vi "ProjectEditInterface.vi"(8 "error in (no error)":errorcluster, 11 "Project.lvclass In":refnum<class "Project.lvclass">) -> (0 "error out":errorcluster, 3 "Project.lvclass Out":refnum<class "Project.lvclass">)   [LabVIEW 2014, in "Project.lvclass"]
uses:
  Project.lvclass
panel:
  in  "ModifyStep":bool
  in  "RemoveStep":bool
  in  "AddStep":bool
  in  "StepList":i32(listbox)
  in  "ProjectList":i32(listbox)
  in  "RemoveProject":bool
  in  "AddProject":bool
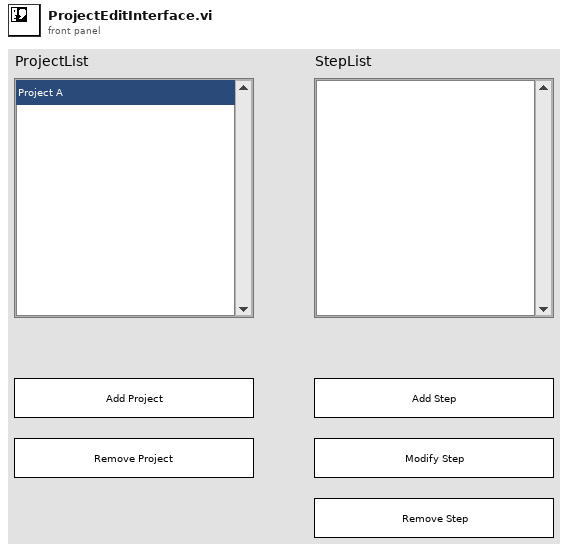
[diagram p1: front panel]
types:
  T1 = typedef "StepData.lvclass/StepTypeEnum.ctl" = enum16{"Move", "Measure"}
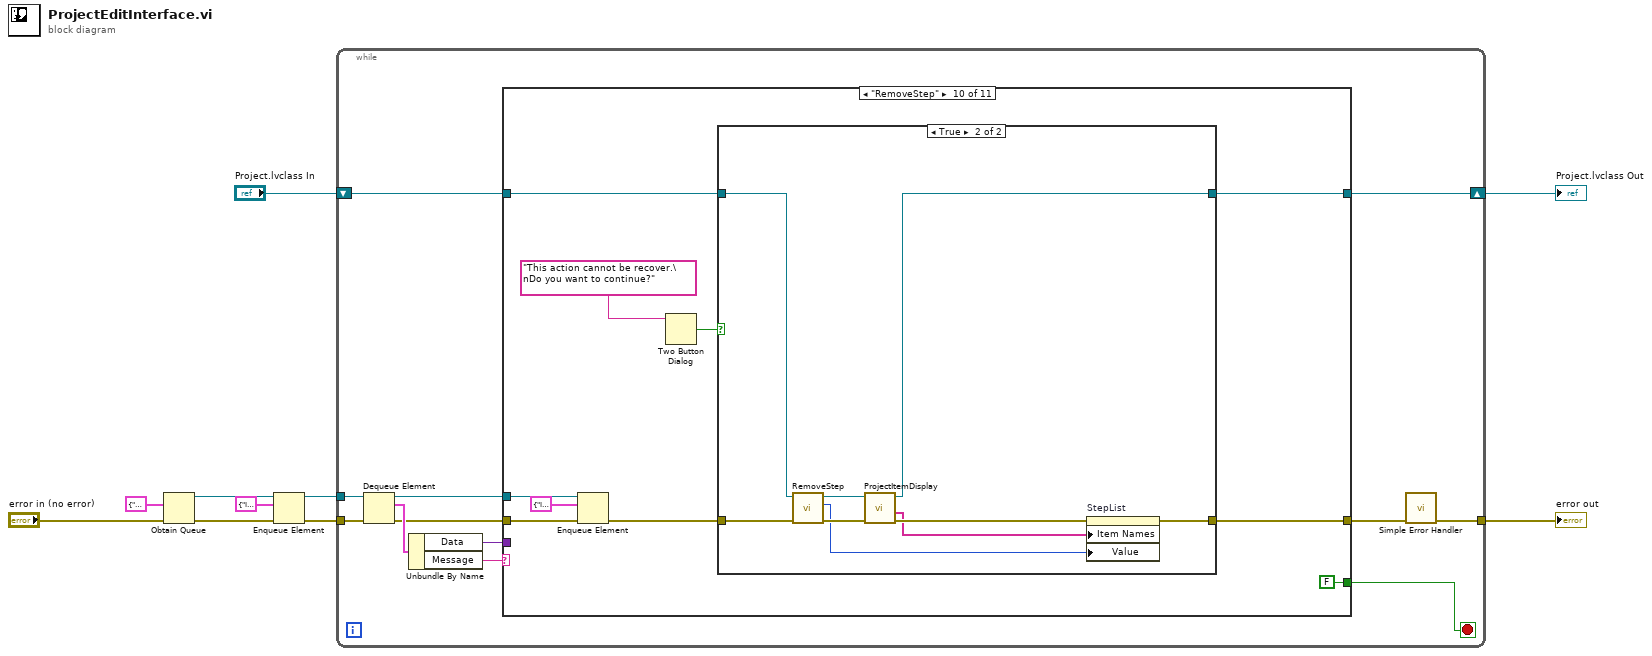
[diagram p0: block diagram]
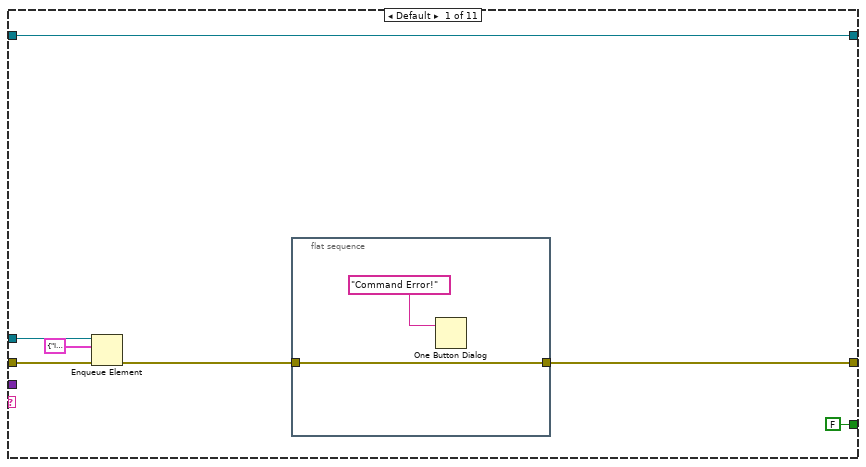
[diagram p2: hidden frame]
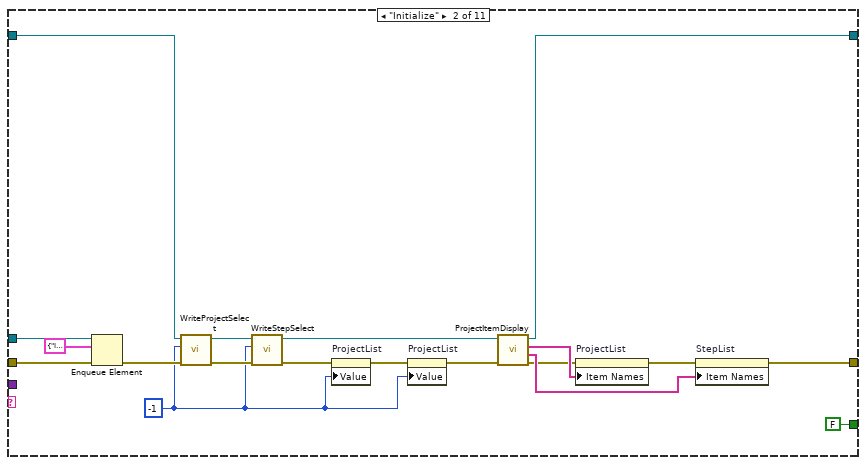
[diagram p3: hidden frame]
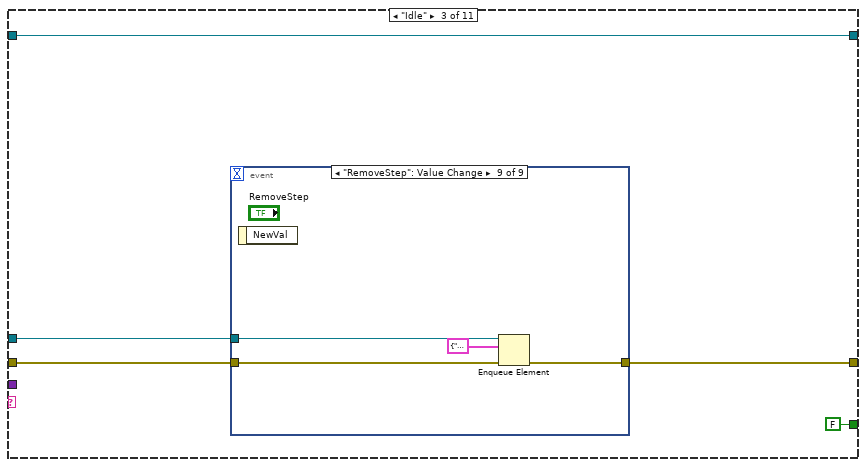
[diagram p4: hidden frame]
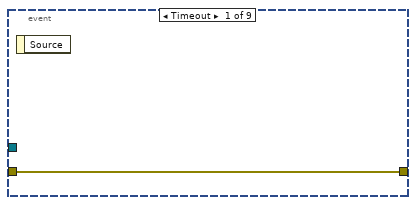
[diagram p5: hidden frame]
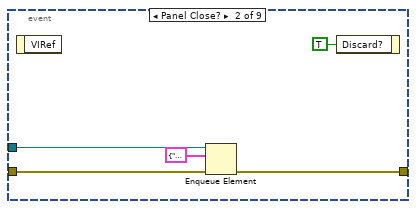
[diagram p6: hidden frame]
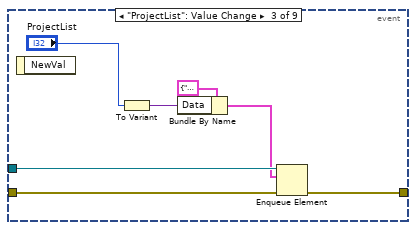
[diagram p7: hidden frame]
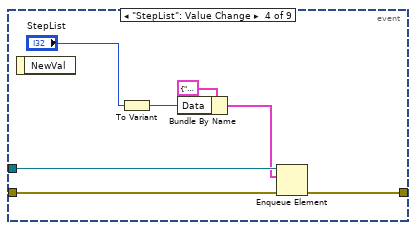
[diagram p8: hidden frame]
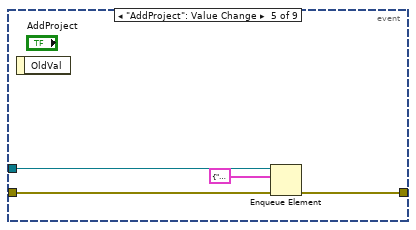
[diagram p9: hidden frame]
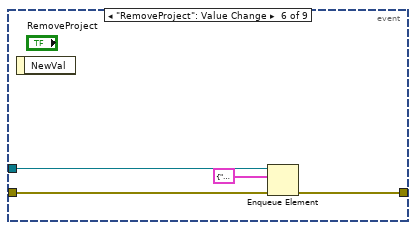
[diagram p10: hidden frame]
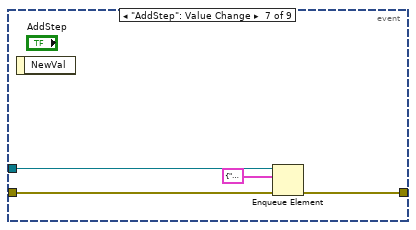
[diagram p11: hidden frame]
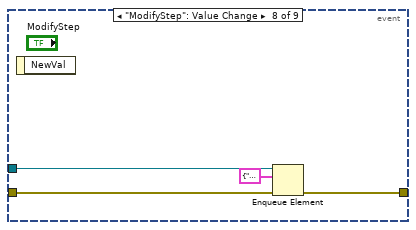
[diagram p12: hidden frame]
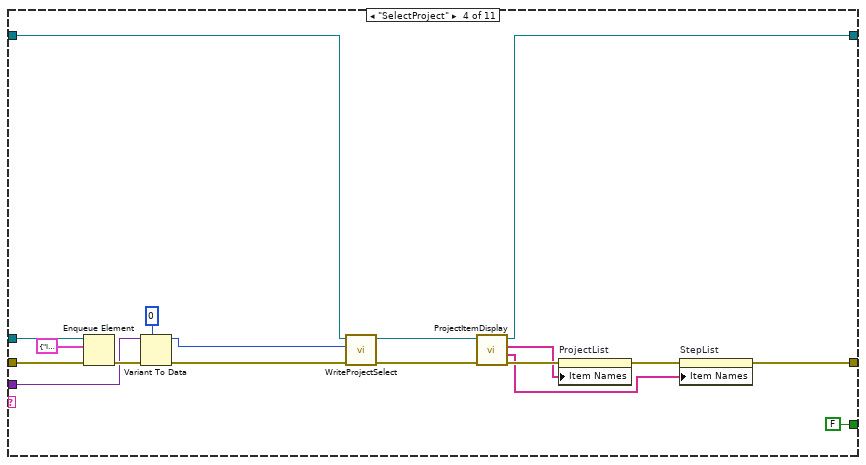
[diagram p13: hidden frame]
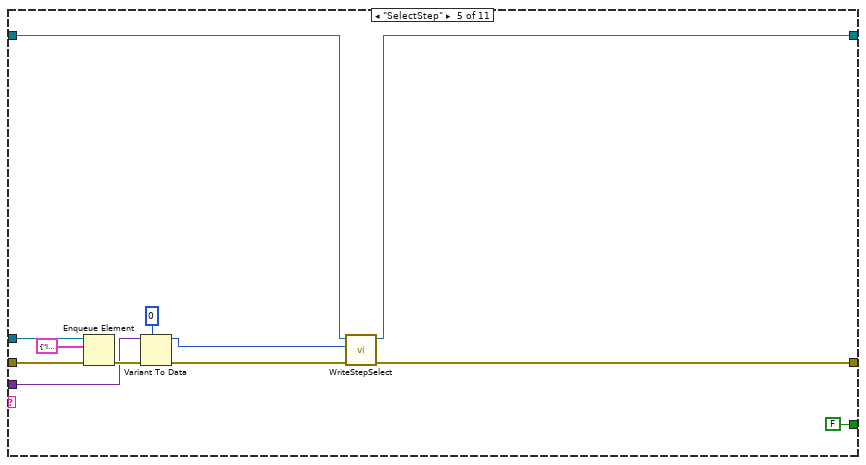
[diagram p14: hidden frame]
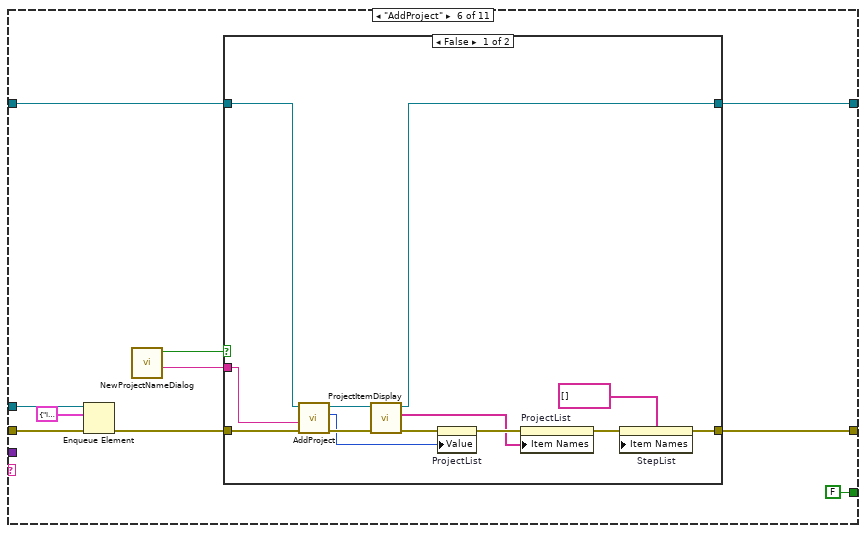
[diagram p15: hidden frame]
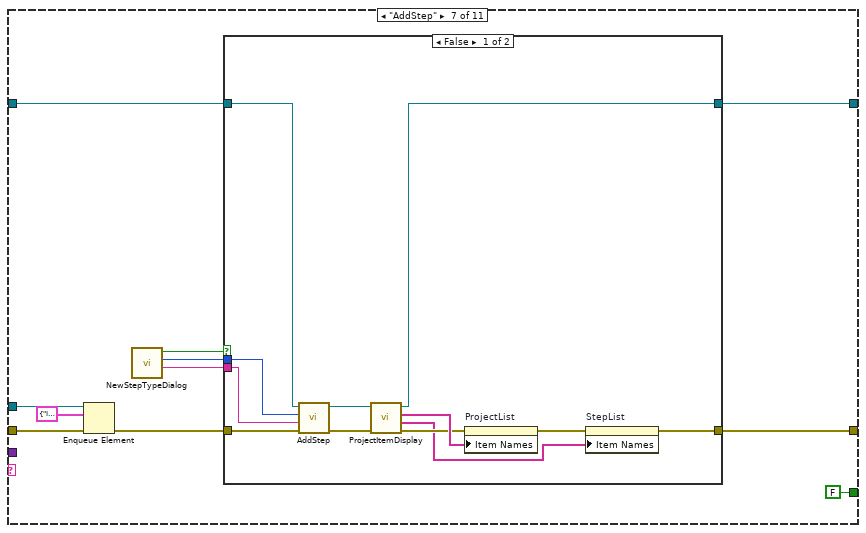
[diagram p17: hidden frame]
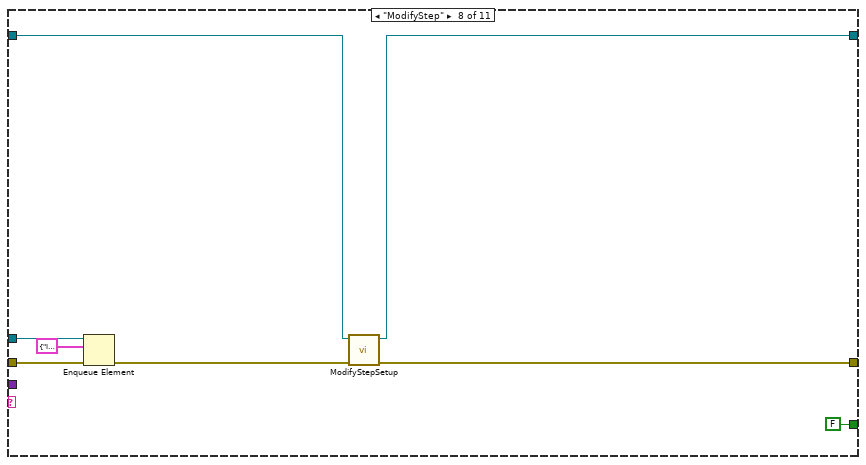
[diagram p19: hidden frame]
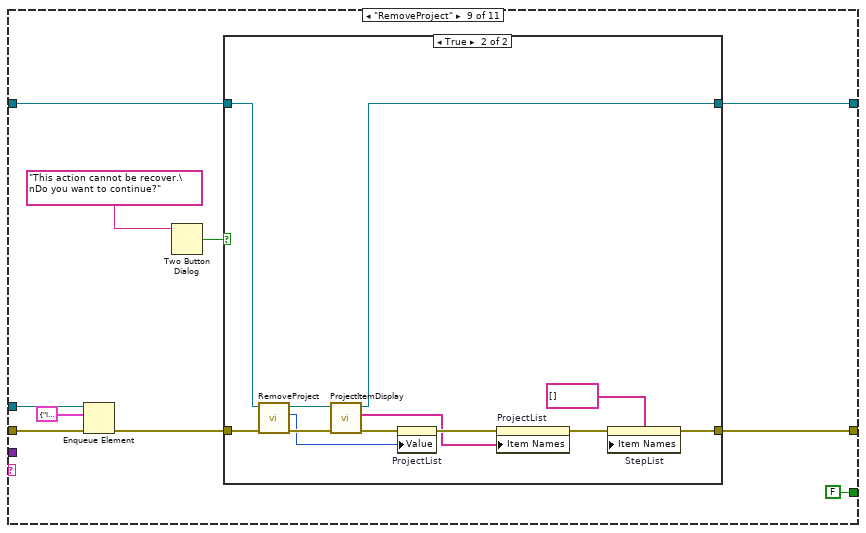
[diagram p20: hidden frame]
diagram:
  n1 = Obtain Queue(element data type=cluster{"Message":string, "Data":variant} {"Message"="", "Data"=variant}, error in (no error)="error in (no error)") -> (queue out=w9:refnum<queue>, error out=w10:errorcluster)  [unwired: 3 in, 1 out]
  n2 = Enqueue Element(queue=w9, element=cluster{"Message":string, "Data":variant} {"Message"="Initialize", "Data"=variant}, error in (no error)=w10) -> (queue out=w6:refnum<queue>, error out=w5:errorcluster)  [unwired: 1 in, 1 out]
  n3 = while {
    tunnel: w6 -> [w22]
    tunnel: w5 -> [w21]
    shift-right: [w14] -> w3
    shift-left: "Project.lvclass In" -> [w13]
    tunnel: [w11] -> w1
    stop <- w15 stop-if-true
    n4 = Dequeue Element(queue=w22, error in (no error)=w21) -> (queue out=w16:refnum<queue>, element=w20:cluster{"Message":string, "Data":variant}, error out=w18:errorcluster)  [unwired: 1 in, 1 out]
    n5 = Unbundle By Name(w20) -> ("Data"=w12:variant, "Message"=w19:string)
    n6 = case shown="\"RemoveStep\"" w19 {
      tunnel: w18 -> [w25 w50 w54 w113 w125 w135 w161 w183 w193 w217 w232]
      tunnel: [w29 w32 w53 w96 w114 w128 w156 w178 w188 w212 w230] -> w17
      tunnel: w16 -> [w23 w49 w55 w112 w124 w134 w160 w182 w192 w216 w231]
      tunnel: [FALSE FALSE FALSE FALSE FALSE FALSE FALSE FALSE FALSE FALSE TRUE] -> w15
      tunnel: [w27 w46 w51 w101 w115 w126 w154 w176 w184 w208 w229] -> w14
      tunnel: w13 -> [w27 w38 w51 w105 w117 w127 w155 w177 w185 w209 w229]
      tunnel: w12 -> [_ _ _ w108 w120 _ _ _ _ _ _]
      frame Default {
        n7 = Enqueue Element(queue=w23, element=cluster{"Message":string, "Data":variant} {"Message"="Idle", "Data"=variant}, error in (no error)=w25) -> (error out=w24:errorcluster)  [unwired: 1 in, 2 out]
        n8 = flat-sequence {
          tunnel: w24 -> [w31]
          tunnel: [w31] -> w29
          frame #0 {
            n9 = One Button Dialog(message="Command Error!") -> ()  [unwired: 1 in, 1 out]
          }
        }
      }
      frame "Initialize" {
        w36 = -1 ("ProjectList")
        n10 = Enqueue Element(queue=w49, element=cluster{"Message":string, "Data":variant} {"Message"="Idle", "Data"=variant}, error in (no error)=w50) -> (error out=w37:errorcluster)  [unwired: 1 in, 2 out]
        n11 = call "WriteProjectSelect.vi"("error in (no error)"=w37, "ProjectSelectIdx"=w36, "Project.lvclass In"=w38) -> ("error out"=w39:errorcluster, "Project.lvclass Out"=w40:refnum<class "Project.lvclass">)  [unwired: 7 in]
        n12 = call "WriteStepSelect.vi"("error in (no error)"=w39, "StepSelectIdx"=w36, "Project.lvclass In"=w40) -> ("error out"=w41:errorcluster, "Project.lvclass Out"=w42:refnum<class "Project.lvclass">)  [unwired: 7 in]
        n13 = property on="ProjectList" class="LstBox (strict)"(error in=w41, "Value"=w36) -> (error out=w44:errorcluster)  [unwired: 1 in, 1 out]
        n14 = property on="ProjectList" class="LstBox (strict)"(error in=w44, "Value"=w36) -> (error out=w43:errorcluster)  [unwired: 1 in, 1 out]
        n15 = call "ProjectItemDisplay.vi"("error in (no error)"=w43, "Project.lvclass In"=w42) -> ("error out"=w34:errorcluster, "StepNames"=w35:string[], "ProjectNames"=w45:string[], "Project.lvclass Out"=w46:refnum<class "Project.lvclass">)  [unwired: 5 in, 1 out]
        n16 = property on="ProjectList" class="LstBox (strict)"(error in=w34, "Item Names"=w45) -> (error out=w33:errorcluster)  [unwired: 1 in, 1 out]
        n17 = property on="StepList" class="LstBox (strict)"(error in=w33, "Item Names"=w35) -> (error out=w32:errorcluster)  [unwired: 1 in, 1 out]
      }
      frame "Idle" {
        n18 = event shown="[8] \"RemoveStep\": Value Change" {
          selector: _ -> [_ _ _ _ _ _ _ _ _]
          dyn-events: _ -> [_ _ _ _ _ _ _ _ _]
          timeout: _ -> [_ _ _ _ _ _ _ _ _]
          tunnel: w55 -> [_ w58 w66 w73 w78 w82 w85 w89 w93]
          tunnel: w54 -> [w56 w60 w68 w75 w79 w83 w87 w91 w95]
          tunnel: [w56 w59 w67 w74 w77 w81 w86 w90 w94] -> w53
          event Timeout {
            n19 = event-data() -> ()  [unwired: 1 in, 1 out]
          }
          event Panel Close? {
            n20 = event-data() -> ()  [unwired: 1 in, 1 out]
            n21 = Enqueue Element(queue=w58, element=cluster{"Message":string, "Data":variant} {"Message"="Exit", "Data"=variant}, error in (no error)=w60) -> (error out=w59:errorcluster)  [unwired: 1 in, 2 out]
            n22 = event-data("Discard?"=TRUE) -> ()  [unwired: 1 in, 1 out]
          }
          event "ProjectList": Value Change {
            n23 = event-data() -> ()  [unwired: 1 in, 1 out]
            n24 = To Variant(anything="ProjectList") -> (Variant=w64:variant)
            n25 = Bundle By Name(cluster=cluster{"Message":string, "Data":variant} {"Message"="SelectProject", "Data"=variant} ("element"), "Data"=w64) -> (w63:cluster{"Message":string, "Data":variant})
            n26 = Enqueue Element(queue=w66, element=w63, error in (no error)=w68) -> (error out=w67:errorcluster)  [unwired: 1 in, 2 out]
          }
          event "StepList": Value Change {
            n27 = event-data() -> ()  [unwired: 1 in, 1 out]
            n28 = To Variant(anything="StepList") -> (Variant=w71:variant)
            n29 = Bundle By Name(cluster=cluster{"Message":string, "Data":variant} {"Message"="SelectStep", "Data"=variant} ("element"), "Data"=w71) -> (w70:cluster{"Message":string, "Data":variant})
            n30 = Enqueue Element(queue=w73, element=w70, error in (no error)=w75) -> (error out=w74:errorcluster)  [unwired: 1 in, 2 out]
          }
          event "AddProject": Value Change {
            n31 = event-data() -> ()  [unwired: 1 in, 1 out]
            n32 = Enqueue Element(queue=w78, element=cluster{"Message":string, "Data":variant} {"Message"="AddProject", "Data"=variant}, error in (no error)=w79) -> (error out=w77:errorcluster)  [unwired: 1 in, 2 out]
          }
          event "RemoveProject": Value Change {
            n33 = event-data() -> ()  [unwired: 1 in, 1 out]
            n34 = Enqueue Element(queue=w82, element=cluster{"Message":string, "Data":variant} {"Message"="RemoveProject", "Data"=variant}, error in (no error)=w83) -> (error out=w81:errorcluster)  [unwired: 1 in, 2 out]
          }
          event "AddStep": Value Change {
            n35 = event-data() -> ()  [unwired: 1 in, 1 out]
            n36 = Enqueue Element(queue=w85, element=cluster{"Message":string, "Data":variant} {"Message"="AddStep", "Data"=variant}, error in (no error)=w87) -> (error out=w86:errorcluster)  [unwired: 1 in, 2 out]
          }
          event "ModifyStep": Value Change {
            n37 = event-data() -> ()  [unwired: 1 in, 1 out]
            n38 = Enqueue Element(queue=w89, element=cluster{"Message":string, "Data":variant} {"Message"="ModifyStep", "Data"=variant}, error in (no error)=w91) -> (error out=w90:errorcluster)  [unwired: 1 in, 2 out]
          }
          event "RemoveStep": Value Change {
            n39 = event-data() -> ()  [unwired: 1 in, 1 out]
            n40 = Enqueue Element(queue=w93, element=cluster{"Message":string, "Data":variant} {"Message"="RemoveStep", "Data"=variant}, error in (no error)=w95) -> (error out=w94:errorcluster)  [unwired: 1 in, 2 out]
          }
        }
      }
      frame "SelectProject" {
        n41 = Enqueue Element(queue=w112, element=cluster{"Message":string, "Data":variant} {"Message"="Idle", "Data"=variant}, error in (no error)=w113) -> (error out=w109:errorcluster)  [unwired: 1 in, 2 out]
        n42 = Variant To Data(error in=w109, type=0, Variant=w108) -> (data=w104:i32, error out=w106:errorcluster)
        n43 = call "WriteProjectSelect.vi"("error in (no error)"=w106, "ProjectSelectIdx"=w104, "Project.lvclass In"=w105) -> ("error out"=w103:errorcluster, "Project.lvclass Out"=w102:refnum<class "Project.lvclass">)  [unwired: 7 in]
        n44 = call "ProjectItemDisplay.vi"("error in (no error)"=w103, "Project.lvclass In"=w102) -> ("error out"=w100:errorcluster, "StepNames"=w97:string[], "ProjectNames"=w98:string[], "Project.lvclass Out"=w101:refnum<class "Project.lvclass">)  [unwired: 5 in, 1 out]
        n45 = property on="ProjectList" class="LstBox (strict)"(error in=w100, "Item Names"=w98) -> (error out=w99:errorcluster)  [unwired: 1 in, 1 out]
        n46 = property on="StepList" class="LstBox (strict)"(error in=w99, "Item Names"=w97) -> (error out=w96:errorcluster)  [unwired: 1 in, 1 out]
      }
      frame "SelectStep" {
        n47 = Enqueue Element(queue=w124, element=cluster{"Message":string, "Data":variant} {"Message"="Idle", "Data"=variant}, error in (no error)=w125) -> (error out=w121:errorcluster)  [unwired: 1 in, 2 out]
        n48 = Variant To Data(error in=w121, type=0, Variant=w120) -> (data=w116:i32, error out=w118:errorcluster)
        n49 = call "WriteStepSelect.vi"("error in (no error)"=w118, "StepSelectIdx"=w116, "Project.lvclass In"=w117) -> ("error out"=w114:errorcluster, "Project.lvclass Out"=w115:refnum<class "Project.lvclass">)  [unwired: 7 in]
      }
      frame "AddProject" {
        n50 = Enqueue Element(queue=w134, element=cluster{"Message":string, "Data":variant} {"Message"="Idle", "Data"=variant}, error in (no error)=w135) -> (error out=w129:errorcluster)  [unwired: 1 in, 2 out]
        n51 = call "NewProjectNameDialog.vi"() -> ("Project Name Out"=w130:string, "Cancel?"=w131:bool)  [unwired: 10 in]
        n52 = case shown="False" w131 {
          tunnel: w130 -> [w139 _]
          tunnel: w129 -> [w148 w150]
          tunnel: [w137 w150] -> w128
          tunnel: w127 -> [w147 w149]
          tunnel: [w141 w149] -> w126
          frame False {
            n53 = call "AddProject.vi"("error in (no error)"=w148, "NewProjectName"=w139, "Project.lvclass In"=w147) -> ("error out"=w146:errorcluster, "ProjectSelectIdx"=w142:i32, "Project.lvclass Out"=w145:refnum<class "Project.lvclass">)  [unwired: 6 in]
            n54 = call "ProjectItemDisplay.vi"("error in (no error)"=w146, "Project.lvclass In"=w145) -> ("error out"=w144:errorcluster, "ProjectNames"=w140:string[], "Project.lvclass Out"=w141:refnum<class "Project.lvclass">)  [unwired: 5 in, 2 out]
            n55 = property on="ProjectList" class="LstBox (strict)"(error in=w144, "Value"=w142) -> (error out=w143:errorcluster)  [unwired: 1 in, 1 out]
            n56 = property on="ProjectList" class="LstBox (strict)"(error in=w143, "Item Names"=w140) -> (error out=w138:errorcluster)  [unwired: 1 in, 1 out]
            n57 = property on="StepList" class="LstBox (strict)"(error in=w138, "Item Names"=string[] []) -> (error out=w137:errorcluster)  [unwired: 1 in, 1 out]
          }
          frame True {
          }
        }
      }
      frame "AddStep" {
        n58 = Enqueue Element(queue=w160, element=cluster{"Message":string, "Data":variant} {"Message"="Idle", "Data"=variant}, error in (no error)=w161) -> (error out=w157:errorcluster)  [unwired: 1 in, 2 out]
        n59 = call "NewStepTypeDialog.vi"() -> ("Step Name Out"=w152:string, "Step Type Out"=w151:T1, "Cancel?"=w153:bool)  [unwired: 9 in]
        n60 = case shown="False" w153 {
          tunnel: w157 -> [w169 w175]
          tunnel: [w163 w175] -> w156
          tunnel: w155 -> [w171 w174]
          tunnel: [w173 w174] -> w154
          tunnel: w152 -> [w167 _]
          tunnel: w151 -> [w165 _]
          frame False {
            n61 = call "AddStep.vi"("error in (no error)"=w169, "StepName"=w167, "StepType"=w165, "Project.lvclass In"=w171) -> ("error out"=w168:errorcluster, "Project.lvclass Out"=w170:refnum<class "Project.lvclass">)  [unwired: 6 in]
            n62 = call "ProjectItemDisplay.vi"("error in (no error)"=w168, "Project.lvclass In"=w170) -> ("error out"=w166:errorcluster, "StepNames"=w162:string[], "ProjectNames"=w172:string[], "Project.lvclass Out"=w173:refnum<class "Project.lvclass">)  [unwired: 5 in, 1 out]
            n63 = property on="ProjectList" class="LstBox (strict)"(error in=w166, "Item Names"=w172) -> (error out=w164:errorcluster)  [unwired: 1 in, 1 out]
            n64 = property on="StepList" class="LstBox (strict)"(error in=w164, "Item Names"=w162) -> (error out=w163:errorcluster)  [unwired: 1 in, 1 out]
          }
          frame True {
          }
        }
      }
      frame "ModifyStep" {
        n65 = Enqueue Element(queue=w182, element=cluster{"Message":string, "Data":variant} {"Message"="Idle", "Data"=variant}, error in (no error)=w183) -> (error out=w179:errorcluster)  [unwired: 1 in, 2 out]
        n66 = call "ModifyStepSetup.vi"("error in (no error)"=w179, "Project.lvclass In"=w177) -> ("error out"=w178:errorcluster, "Project.lvclass Out"=w176:refnum<class "Project.lvclass">)  [unwired: 8 in]
      }
      frame "RemoveProject" {
        n67 = Enqueue Element(queue=w192, element=cluster{"Message":string, "Data":variant} {"Message"="Idle", "Data"=variant}, error in (no error)=w193) -> (error out=w189:errorcluster)  [unwired: 1 in, 2 out]
        n68 = Two Button Dialog(message="This action cannot be recover.\nDo you want to continue?") -> (T button?=w187:bool)  [unwired: 2 in]
        n69 = case shown="True" w187 {
          tunnel: w189 -> [w195 w204]
          tunnel: [w195 w197] -> w188
          tunnel: w185 -> [w194 w200]
          tunnel: [w194 w199] -> w184
          frame False {
          }
          frame True {
            n70 = call "RemoveProject.vi"("error in (no error)"=w204, "Project.lvclass In"=w200) -> ("error out"=w203:errorcluster, "ProjectSelectIdx"=w202:i32, "Project.lvclass Out"=w201:refnum<class "Project.lvclass">)  [unwired: 7 in]
            n71 = call "ProjectItemDisplay.vi"("error in (no error)"=w203, "Project.lvclass In"=w201) -> ("error out"=w207:errorcluster, "ProjectNames"=w205:string[], "Project.lvclass Out"=w199:refnum<class "Project.lvclass">)  [unwired: 5 in, 2 out]
            n72 = property on="ProjectList" class="LstBox (strict)"(error in=w207, "Value"=w202) -> (error out=w206:errorcluster)  [unwired: 1 in, 1 out]
            n73 = property on="ProjectList" class="LstBox (strict)"(error in=w206, "Item Names"=w205) -> (error out=w198:errorcluster)  [unwired: 1 in, 1 out]
            n74 = property on="StepList" class="LstBox (strict)"(error in=w198, "Item Names"=string[] []) -> (error out=w197:errorcluster)  [unwired: 1 in, 1 out]
          }
        }
      }
      frame "RemoveStep" {
        n75 = Enqueue Element(queue=w216, element=cluster{"Message":string, "Data":variant} {"Message"="Idle", "Data"=variant}, error in (no error)=w217) -> (error out=w213:errorcluster)  [unwired: 1 in, 2 out]
        n76 = Two Button Dialog(message="This action cannot be recover.\nDo you want to continue?") -> (T button?=w211:bool)  [unwired: 2 in]
        n77 = case shown="True" w211 {
          tunnel: w213 -> [w219 w223]
          tunnel: [w219 w228] -> w212
          tunnel: w209 -> [w218 w226]
          tunnel: [w218 w227] -> w208
          frame False {
          }
          frame True {
            n78 = call "RemoveStep.vi"("error in (no error)"=w223, "Project.lvclass In"=w226) -> ("error out"=w224:errorcluster, "StepIdx"=w220:i32, "Project.lvclass Out"=w225:refnum<class "Project.lvclass">)  [unwired: 7 in]
            n79 = call "ProjectItemDisplay.vi"("error in (no error)"=w224, "Project.lvclass In"=w225) -> ("error out"=w222:errorcluster, "StepNames"=w221:string[], "Project.lvclass Out"=w227:refnum<class "Project.lvclass">)  [unwired: 5 in, 2 out]
            n80 = property on="StepList" class="LstBox (strict)"(error in=w222, "Item Names"=w221, "Value"=w220) -> (error out=w228:errorcluster)  [unwired: 1 in, 1 out]
          }
        }
      }
      frame "Exit" {
        n81 = Release Queue(queue=w231, error in (no error)=w232) -> (error out=w230:errorcluster)  [unwired: 1 in, 2 out]
      }
    }
    n82 = call <vilib>:"Simple Error Handler.vi"("error in (no error)"=w17) -> ("error out"=w11:errorcluster)  [unwired: 4 in, 4 out]
  }
  "Project.lvclass Out" <- w3
  "error out" <- w1
